vi "Read Best Cost.vi"(8 "error in (no error)":errorcluster, 11 "State Value in":refnum<class "State Value.lvclass">) -> (0 "error out":errorcluster, 2 "Best Cost":u64, 3 "State Value out":refnum<class "State Value.lvclass">)   [LabVIEW 2019, in "23.lvlib" / "State Value.lvclass"]
uses:
  State Value.lvclass
  State Value.lvclass/State Value.ctl
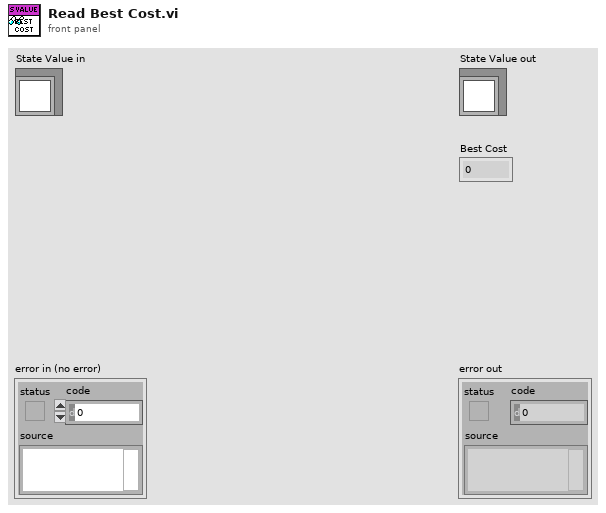
[diagram p1: front panel]
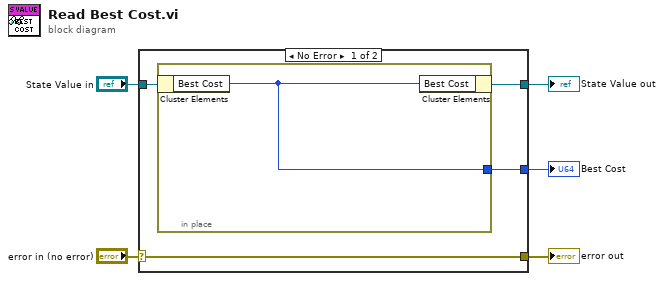
[diagram p0: block diagram]
diagram:
  n1 = case shown="No Error" "error in (no error)" {
    selector: "error in (no error)" -> [w9 w11]
    tunnel: [w9 w11] -> w4
    tunnel: [w6 w12] -> w2
    tunnel: "State Value in" -> [w7 w12]
    tunnel: [w8 _] -> w1
    frame No Error {
      n2 = in-place {
        in-place-border: [w10] -> w8
        n3 = in-place-cluster #1(w7) -> ("Best Cost"=w10:u64)
        n4 = in-place-cluster #1("Best Cost"=w10) -> (w6:refnum<class "State Value.lvclass">)
      }
    }
    frame Error {
    }
  }
  "error out" <- w4
  "State Value out" <- w2
  "Best Cost" <- w1
